vi "FSR_4_SENSOR_FSR_final.vi"() -> ()   [LabVIEW 2013]
uses:
  D:/Program Files (x86)/National Instruments/LabVIEW 2013/examples/Instrument IO/Serial/support/Serial - Settings.ctl
  <vilib>/Instr/_visa.llb/VISA Configure Serial Port (Instr).vi
panel:
  in  "Boolean":bool
  out "Waveform Chart":dynamicdata(graph)
  out "FSR1 Graph":i32(graph)
  out "FSR2Graph":i32(graph)
  out "FSR3Graph":i32(graph)
  out "FSR1 Gauge":dbl(knob) scale=0.0..10.0
  out "FSR2 Gauge":dbl(knob) scale=0.0..10.0
  out "FSR3 Gauge":dbl(knob) scale=0.0..10.0
  out "FSR1":string
  out "FSR2":string
  out "FSR3":string
  out "FSR4 Gauge":dbl(knob) scale=0.0..1200.0
  in  "stop":bool
  out "FSR4 Graph":i32(graph)
  out "FSR4":string
  out "read buffer":string
  in  "byte count":u32
  in  "Serial Settings":T1={"baud rate"=9600, "data bits"=8, "parity"=enum."None", "stop bits"=10, "flow control"=0} {"flow control" items=["None"=0, "XON/XOFF"=1, "RTS/CTS"=2, "DTR/DSR"=4]; "stop bits" items=["1.0"=10, "1.5"=15, "2.0"=20]; "data bits" min=5 max=8 step=1; "baud rate" items=["75"=75, "110"=110, "134"=134, "150"=150, "300"=300, "600"=600, "1200"=1200, "1800"=1800, "2400"=2400, "4800"=4800, "7200"=7200, "9600"=9600, "14400"=14400, "19200"=19200, "28800"=28800, "38400"=38400, "56000"=56000, "57600"=57600, "115200"=115200, "128000"=128000, "230400"=230400]}
  in  "VISA resource name":refnum<visa-resource-name>
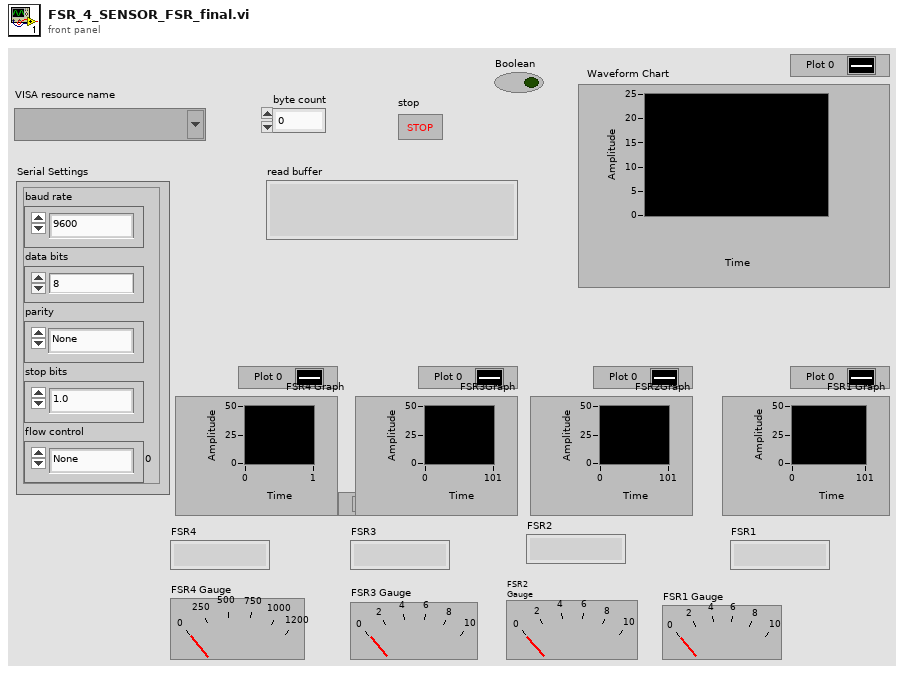
[diagram p1: front panel]
types:
  T1 = typedef "Serial - Settings.ctl" = cluster{"baud rate":u32, "data bits":u16, "parity":enum16{"None", "Odd", "Even", "Mark", "Space"}, "stop bits":u16, "flow control":u16}
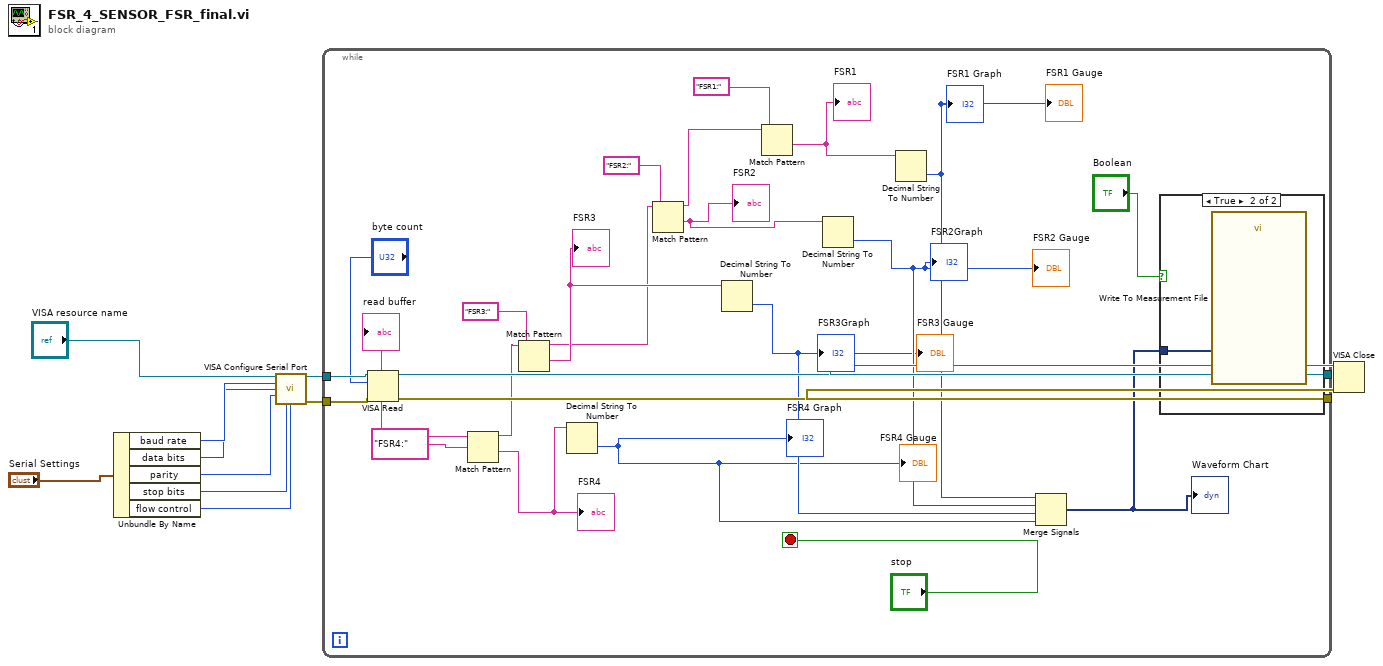
[diagram p0: block diagram]
diagram:
  n1 = Unbundle By Name("Serial Settings") -> ("baud rate"=w9:u32, "data bits"=w8:u16, "parity"=w7:enum16{"None", "Odd", "Even", "Mark", "Space"}, "stop bits"=w6:u16, "flow control"=w5:u16)
  n2 = call-poly "VISA Configure Serial Port"("VISA resource name"="VISA resource name", "baud rate (9600)"=w9, "data bits (8)"=w8, "parity (0:none)"=w7, "stop bits (10: 1 bit)"=w6, "flow control (0:none)"=w5) -> ("VISA resource name out"=w4:refnum<visa-resource-name>, "error out"=w3:errorcluster)  [unwired: 8 in]
  n3 = while {
    tunnel: w4 -> [w35]
    tunnel: w3 -> [w34]
    tunnel: [w29] -> w2
    tunnel: [w28] -> w1
    stop <- "stop" stop-if-true
    n4 = VISA Read(VISA resource name=w35, byte count="byte count", error in (no error)=w34) -> (VISA resource name out=w28:refnum<visa-resource-name>, read buffer=w32:string, error out=w29:errorcluster)  [unwired: 1 out]
    "read buffer" <- w32
    n5 = Match Pattern(string=w32, regular expression="FSR4:") -> (before substring=w27:string, after substring=w30:string)  [unwired: 1 in, 2 out]
    "FSR4" <- w30
    n6 = Match Pattern(string=w27, regular expression="FSR3:") -> (before substring=w19:string, after substring=w22:string)  [unwired: 1 in, 2 out]
    "FSR3" <- w22
    n7 = Decimal String To Number(string=w30) -> (number=w13:i32)  [unwired: 2 in, 1 out]
    "FSR4 Graph" <- w13
    "FSR4 Gauge" <- w13
    n8 = Match Pattern(string=w19, regular expression="FSR2:") -> (before substring=w26:string, after substring=w21:string)  [unwired: 1 in, 2 out]
    "FSR2" <- w21
    n9 = Decimal String To Number(string=w22) -> (number=w14:i32)  [unwired: 2 in, 1 out]
    "FSR3 Gauge" <- w14
    "FSR3Graph" <- w14
    n10 = Match Pattern(string=w26, regular expression="FSR1:") -> (after substring=w20:string)  [unwired: 1 in, 3 out]
    "FSR1" <- w20
    n11 = Decimal String To Number(string=w21) -> (number=w15:i32)  [unwired: 2 in, 1 out]
    "FSR2 Gauge" <- w15
    "FSR2Graph" <- w15
    n12 = Decimal String To Number(string=w20) -> (number=w16:i32)  [unwired: 2 in, 1 out]
    "FSR1 Gauge" <- w16
    "FSR1 Graph" <- w16
    n13 = Merge Signals "Merge Signals"(w16, w15, w14, w13) -> (w12:dynamicdata)
    "Waveform Chart" <- w12
    n14 = case shown="True" "Boolean" {
      tunnel: w12 -> [_ w36]
      frame False {
      }
      frame True {
        n15 = call "Write To Measurement File"("Signals"=w36) -> ()  [unwired: 16 in, 3 out]
      }
    }
  }
  n16 = VISA Close(VISA resource name=w1, error in (no error)=w2) -> ()  [unwired: 1 out]
